vi "001write_file.vi"() -> ()   [LabVIEW 2012]
panel:
  in  "停止 2":bool
  in  "停止":bool
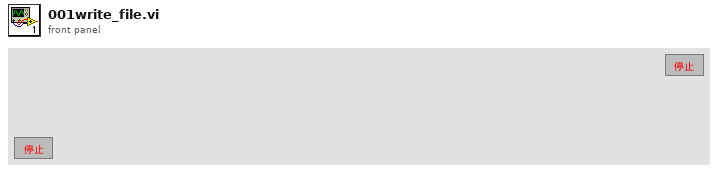
[diagram p1: front panel]
types:
  T1 = enum16{"open", "replace", "create", "open or create", "replace or create", "replace or create with confirmation"}
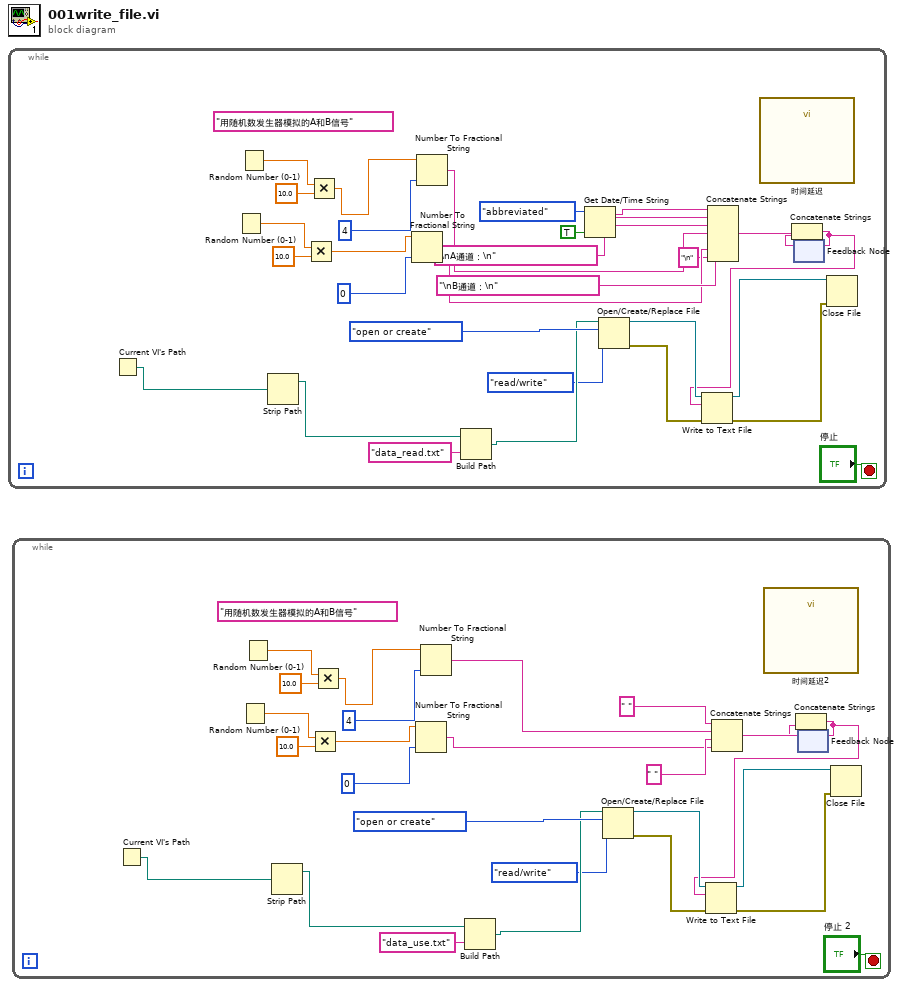
[diagram p0: block diagram]
diagram:
  n1 = while {
    stop <- "停止" stop-if-true
    (unwired) "用随机数发生器模拟的A和B信号"
    n2 = Current VI's Path() -> (path=w30:path)
    n3 = Random Number (0-1)() -> (number: 0 to 1=w18:dbl)
    n4 = Random Number (0-1)() -> (number: 0 to 1=w20:dbl)
    n5 = Strip Path(path=w30) -> (stripped path=w29:path)  [unwired: 1 out]
    n6 = Multiply(x=w18, y=10.0) -> (x*y=w11:dbl)
    n7 = Multiply(x=w20, y=10.0) -> (x*y=w13:dbl)
    n8 = Number To Fractional String(number=w11, precision (6)=i16 0 ("宽度(-)")) -> (F-format string=w5:string)  [unwired: 2 in]
    n9 = Number To Fractional String(number=w13, precision (6)=i16 4 ("宽度(-)")) -> (F-format string=w6:string)  [unwired: 2 in]
    n10 = Build Path(base path=w29, name or relative path="data_read.txt" ("名称或相对路径")) -> (appended path=w24:path)
    n11 = Get Date/Time String(date format (0)=enum16{"short", "long", "abbreviated"}."abbreviated" ("日期格式(0)"), want seconds? (F)=TRUE ("需要秒？(F)")) -> (date string=w27:string, time string=w8:string)  [unwired: 1 in]
    n12 = Open/Create/Replace File(file path (use dialog)=w24, operation (0:open)=T1."open or create" ("操作(0:open)"), access (0:read/write)=enum16{"read/write", "read-only", "write-only"}."read/write" ("权限(0:read/write)")) -> (refnum out=w17:refnum<file>, error out=w14:errorcluster)  [unwired: 3 in, 1 out]
    n13 = Concatenate Strings(w27, w8, "\nA通道：\n" ("字符串"), w6, "\nB通道：\n" ("字符串"), w5, "\n" ("字符串")) -> (w4:string)
    n14 = call "时间延迟"() -> ()  [unwired: 11 in, 1 out]
    n15 = feedback #1() -> (w3:string)  [unwired: 1 in]
    n16 = Concatenate Strings(w4, w3) -> (w2:string)
    n17 = Write to Text File(file (use dialog)=w17, text=w2, error in=w14) -> (refnum out=w16:refnum<file>, error out=w15:errorcluster)  [unwired: 1 in, 1 out]
    n18 = feedback-in #1(w2) -> ()
    n19 = Close File(refnum=w16, error in=w15) -> ()  [unwired: 2 out]
  }
  n20 = while {
    stop <- "停止 2" stop-if-true
    (unwired) "用随机数发生器模拟的A和B信号"
    n21 = Current VI's Path() -> (path=w56:path)
    n22 = Random Number (0-1)() -> (number: 0 to 1=w47:dbl)
    n23 = Random Number (0-1)() -> (number: 0 to 1=w49:dbl)
    n24 = Strip Path(path=w56) -> (stripped path=w55:path)  [unwired: 1 out]
    n25 = Multiply(x=w47, y=10.0) -> (x*y=w40:dbl)
    n26 = Multiply(x=w49, y=10.0) -> (x*y=w42:dbl)
    n27 = Number To Fractional String(number=w40, precision (6)=i16 0 ("宽度(-)")) -> (F-format string=w32:string)  [unwired: 2 in]
    n28 = Number To Fractional String(number=w42, precision (6)=i16 4 ("宽度(-)")) -> (F-format string=w34:string)  [unwired: 2 in]
    n29 = Build Path(base path=w55, name or relative path="data_use.txt" ("名称或相对路径")) -> (appended path=w53:path)
    n30 = Open/Create/Replace File(file path (use dialog)=w53, operation (0:open)=T1."open or create" ("操作(0:open)"), access (0:read/write)=enum16{"read/write", "read-only", "write-only"}."read/write" ("权限(0:read/write)")) -> (refnum out=w46:refnum<file>, error out=w43:errorcluster)  [unwired: 3 in, 1 out]
    n31 = Concatenate Strings(" " ("字符串"), w34, " " ("字符串"), w32) -> (w38:string)
    n32 = call "时间延迟2"() -> ()  [unwired: 11 in, 1 out]
    n33 = feedback #2() -> (w37:string)  [unwired: 1 in]
    n34 = Concatenate Strings(w38, w37) -> (w36:string)
    n35 = Write to Text File(file (use dialog)=w46, text=w36, error in=w43) -> (refnum out=w45:refnum<file>, error out=w44:errorcluster)  [unwired: 1 in, 1 out]
    n36 = feedback-in #2(w36) -> ()
    n37 = Close File(refnum=w45, error in=w44) -> ()  [unwired: 2 out]
  }
